vi "List tables.vi"(8 "error in (no error)":errorcluster, 11 "database":string="database1.mdb") -> (0 "error out":errorcluster, 3 "tables":string[](array[string]))   [LabVIEW 2016, in "数据查询.lvlib"]
uses:
  <vilib>/addons/database/Connection.llb/DB Tools Open Connec (String).vi
  <userlib>/_LVST/sqlite_api/Core/Tables/SQLite_List Tables.vi
  <vilib>/addons/database/NI_Database_API.lvlib
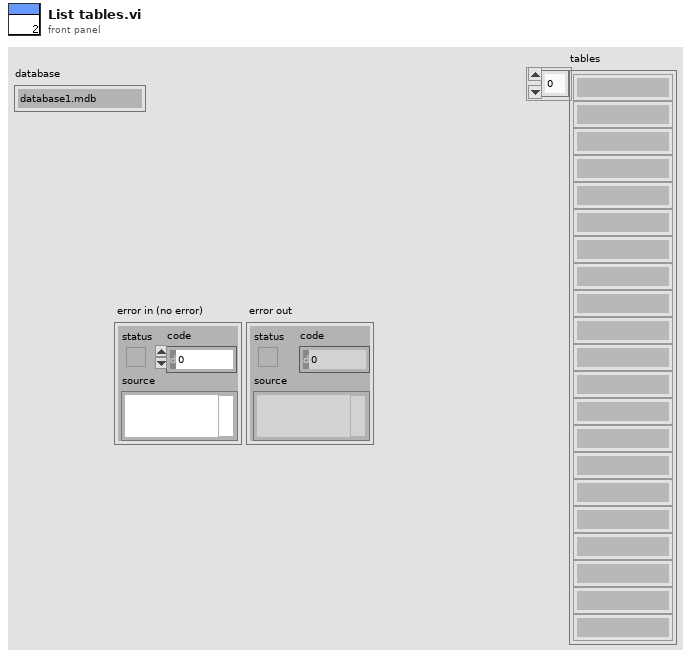
[diagram p1: front panel]
types:
  T1 = typedef "数据库类型.ctl" = enum16{"Access", "SQLite"}
  T2 = typedef "NI_Database_API.lvlib/Conn ObjectReference.ctl" = refnum<k1>
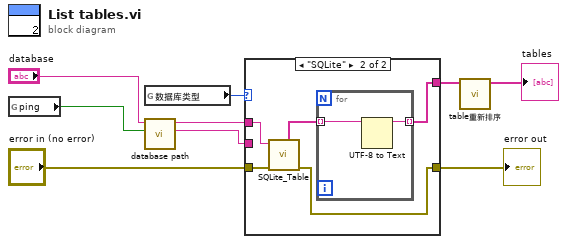
[diagram p0: block diagram]
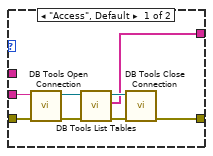
[diagram p2: hidden frame]
diagram:
  n1 = global read "全局变量.vi" "ping"() -> (w3:bool)
  n2 = global read "外部调用接口全局变量.vi" "数据库类型"() -> (w1:T1)
  n3 = call "database path.vi"("ping"=w3, "database"="database") -> ("Connection information"=w2:string, "Path out"=w4:string)  [unwired: 8 in]
  n4 = case shown="\"SQLite\"" w1 {
    tunnel: "error in (no error)" -> [w13 w21]
    tunnel: [w12 w22] -> w8
    tunnel: [w11 w19] -> w7
    tunnel: w4 -> [_ w18]
    tunnel: w2 -> [w10 _]
    frame "Access", Default {
      n5 = call-poly <vilib>:"DB Tools Open Connection.vi"("error in (no error)"=w13, "connection information"=w10) -> ("error out"=w15:errorcluster, "connection reference"=w17:T2)  [unwired: 6 in]
      n6 = call <vilib>:"DB Tools List Tables.vi"("error in (no error)"=w15, "connection reference"=w17) -> ("error out"=w14:errorcluster, "tables"=w11:string[], "connection reference out"=w16:T2)  [unwired: 3 in]
      n7 = call <vilib>:"DB Tools Close Connection.vi"("error in (no error)"=w14, "connection reference"=w16) -> ("error out"=w12:errorcluster)  [unwired: 5 in]
    }
    frame "SQLite" {
      n8 = call-poly <userlib>:"SQLite_Table.vi"("DB Path"=w18, "error in (no error)"=w21) -> ("Tables"=w20:string[], "error out"=w22:errorcluster)  [unwired: 6 in, 1 out]
      n9 = for {
        tunnel: w20 -> [w24] mode=indexing
        tunnel: [w23] -> w19 mode=indexing
        n10 = UTF-8 to Text(11:w24) -> (3:w23:string)  [unwired: 2 in, 1 out]
      }
    }
  }
  "error out" <- w8
  n11 = call "table重新排序.vi"("tables"=w7) -> ("sorted elements"=→"tables":string[])  [unwired: 10 in]
